vi "SphereConvert.vi"(2 "x,y,z in":dbl[](array[numeric]) format="%.2f", 3 "spherical in":dbl[](array[numeric]) format="%.2f", 4 "xyz ?":bool) -> (0 "x,y,z":dbl[](array[numeric]) format="%.2f", 1 "spherical":dbl[](array[numeric]) format="%.2f")   [LabVIEW 2022 SP3]
panel:
  # "transfrom rectangular coordinates to spherical\n\nor spehrical coordinates to rectangular."
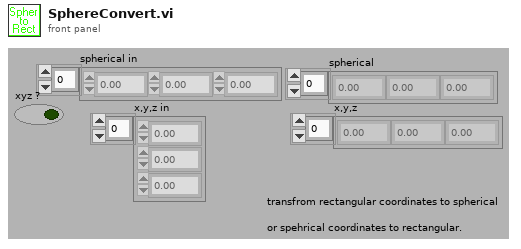
[diagram p1: front panel]
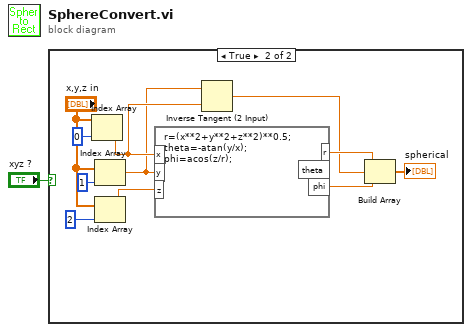
[diagram p0: block diagram]
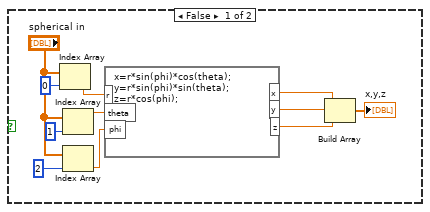
[diagram p2: hidden frame]
diagram:
  n1 = case shown="True" "xyz ?" {
    frame False {
      n2 = Index Array(array="spherical in", index=0 ("Index")) -> (element=w4:dbl)
      n3 = Index Array(array="spherical in", index=1) -> (element=w3:dbl)
      n4 = Index Array(array="spherical in", index=2) -> (element=w2:dbl)
      n5 = formula code="x=r*sin(phi)*cos(theta);\ny=r*sin(phi)*sin(theta);\nz=r*cos(phi);"("r"=w4, "theta"=w3, "phi"=w2) -> ("x"=w12:dbl, "y"=w11:dbl, "z"=w10:dbl)
      n6 = Build Array(w12, w11, w10) -> (→"x,y,z":dbl[])
    }
    frame True {
      n7 = Index Array(array="x,y,z in", index=0 ("Index")) -> (element=w15:dbl)
      n8 = Index Array(array="x,y,z in", index=1) -> (element=w14:dbl)
      n9 = Index Array(array="x,y,z in", index=2) -> (element=w17:dbl)
      n10 = formula code="r=(x**2+y**2+z**2)**0.5;\ntheta=-atan(y/x);\nphi=acos(z/r);"("x"=w15, "y"=w14, "z"=w17) -> ("r"=w23:dbl, "phi"=w22:dbl)  [unwired: 1 out]
      n11 = Inverse Tangent (2 Input)(1:w15, 2:w14) -> (0:w13:dbl)
      n12 = Build Array(w23, w13, w22) -> (→"spherical":dbl[])
    }
  }
